vi "Construct Actor Message Transport.vi"(7 "Return Priority (Normal)":T1=enum."Normal", 9 "Datum Name":string, 10 "Notification Msg":refnum<class "Notification Msg.lvclass">, 11 "Message Enqueuer in":refnum<class "Message Enqueuer.lvclass">) -> (0 "error out":errorcluster, 3 "ActorMessageTransport":refnum<class "ActorMessageTransport.lvclass">)   [LabVIEW 2018, in "MVA Framework.lvlib" / "ActorMessageTransport.lvlib" / "ActorMessageTransport.lvclass"]
doc: "构建Actor消息传输"
uses:
  ActorMessageTransport.lvclass
  <vilib>/ActorFramework/Message Enqueuer/Message Enqueuer.lvclass
  <vilib>/ErrorRing/Error Ring.xnode
  <vilib>/Utility/error.llb/Error Cluster From Error Code.vi
  Notification Msg/Notification Msg.lvclass
  <vilib>/ActorFramework/Message Enqueuer/Message Priority.ctl
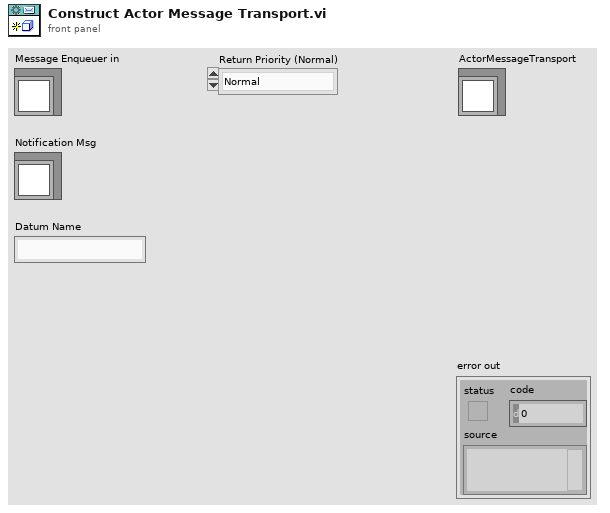
[diagram p1: front panel]
types:
  T1 = typedef "Actor Framework.lvlib/Message Enqueuer.lvclass/Message Priority.ctl" = enum16{"Low", "Normal", "High"}
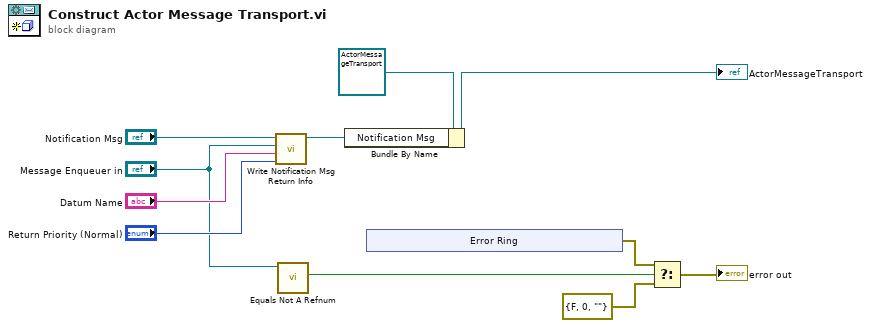
[diagram p0: block diagram]
diagram:
  n1 = call-dynamic "Write Notification Msg Return Info.vi"("Return Priority (Normal)"="Return Priority (Normal)", "Datum Name"="Datum Name", "Message Enqueuer in"="Message Enqueuer in", "Notification Msg In"="Notification Msg") -> ("Notification Msg Out"=w8:refnum<class "Notification Msg.lvclass">)  [unwired: 7 in]
  n2 = call <vilib>:"Equals Not A Refnum.vi"("Message Enqueuer"="Message Enqueuer in") -> ("Not a refnum?"=w4:bool)  [unwired: 10 in]
  n3 = Bundle By Name(cluster=refnum<class "ActorMessageTransport.lvclass"> refnum ("ActorMessageTransport.lvlib:ActorMessageTransport.lvclass"), "Notification Msg"=w8) -> (→"ActorMessageTransport":refnum<class "ActorMessageTransport.lvclass">)
  n4 = xnode "Error Ring"() -> ("错误输出"=w2:errorcluster)
  n5 = Select(t=w2, s=w4, f=errorcluster {"status"=FALSE, "code"=0, "source"=""} ("error constant")) -> (s? t:f=→"error out":errorcluster)
